vi "calc_phasemap_from_stored_images_ec.vi"() -> ()   [LabVIEW 2011]
uses:
  global_vars.vi
  <userlib>/_OpenG.lib/file/file.llb/Build Path - Traditional__ogtk.vi
panel:
  out "Intensity Graph":dbl[][](graph)
  out "u8_ar_phase map 2":u8[][](array[numeric])
  out "df_ar_unwrapped_px_ar 2":dbl[][](array[numeric])
  out "df_ar_unwrapped_px_ar":dbl[][](array[numeric])
  in  "current image 3":string="fringe2"
  out "difference":T1(plugin-control)
  out "Ndist_img":u8[][][](array[numeric])
  in  "read files no-dist":bool
  in  "normalize":bool
  out "Phase Line (unwrapped)":dbl[](graph)=[64.0, 65.0, 66.0, 68.0, 69.0, 70.0, 71.0, 73.0, 74.0, 75.0, 77.0, 78.0, 79.0, 80.0, 81.0, 83.0, 84.0, 85.0, 87.0, 88.0, 89.0, 90.0, 92.0, 93.0, 95.0, 96.0, 97.0, 98.0, 99.0, 101.0, 102.0, 103.0, 104.0, 106.0, 107.0, 108.0, 110.0, 111.0, 112.0, 114.0, 115.0, 116.0, 117.0, 119.0, 120.0, 121.0, 122.0, 124.0, 125.0, 126.0, 128.0, 129.0, 130.0, 131.0, 133.0, 134.0, 135.0, 136.0, 138.0, 139.0, 140.0, 141.0, 143.0, 144.0, 145.0, 147.0, 148.0, 149.0, 151.0, 152.0, 153.0, 154.0, 156.0, 157.0, 158.0, 159.0, 160.0, 162.0, 163.0, 165.0, 166.0, 167.0, 168.0, 170.0, 171.0, 172.0, 174.0, 175.0, 176.0, 177.0, 178.0, 180.0, 181.0, 182.0, 184.0, 185.0, 186.0, 187.0, 189.0, 190.0, 191.0, 193.0, 194.0, 195.0, 196.0, 198.0, 199.0, 200.0, 201.0, 203.0, 204.0, 205.0, 207.0, 208.0, 209.0, 210.0, 212.0, 213.0, 214.0, 215.0, 217.0, 218.0, 219.0, 221.0, 222.0, 223.0, 224.0, 226.0, 227.0, 228.0, 230.0, 231.0, 232.0, 233.0, 234.0, 236.0, 237.0, 238.0, 240.0, 241.0, 242.0, 243.0, 245.0, 246.0, 247.0, 249.0, 250.0, 251.0, 252.0, 254.0, 254.0, 255.0, 257.0, 258.0, 259.0, 260.0, 262.0, 263.0, 264.0, 266.0, 267.0, 268.0, 269.0, 271.0, 272.0, 273.0, 275.0, 276.0, 277.0, 278.0, 279.0, 281.0, 282.0, 283.0, 285.0, 286.0, 287.0, 288.0, 290.0, 291.0, 292.0, 294.0, 295.0, 296.0, 297.0, 299.0, 300.0, 301.0, 302.0, 304.0, 305.0, 306.0, 308.0, 309.0, 310.0, 311.0, 313.0, 314.0, 315.0, 316.0, 318.0, 319.0, 320.0, 322.0, 323.0, 324.0, 325.0, 327.0, 328.0, 329.0, 331.0, 332.0, 333.0, 334.0, 335.0, 337.0, 338.0, 339.0, 341.0, 342.0, 343.0, 344.0, 346.0, 347.0, 349.0, 350.0, 351.0, 352.0, 353.0, 355.0, 356.0, 357.0, 358.0, 360.0, 361.0, 362.0, 364.0, 365.0, 366.0, 368.0, 369.0, 370.0, 371.0, 373.0, 374.0, 375.0, 376.0, 378.0, 379.0, 380.0, 382.0, 383.0, 384.0, 385.0, 387.0, 388.0, 389.0, 390.0, 392.0, 393.0, 394.0, 395.0, 397.0, 398.0, 399.0, 401.0, 402.0, 403.0, 405.0, 406.0, 407.0, 408.0, 410.0, 411.0, 412.0, 413.0, 414.0, 416.0, 417.0, 419.0, 420.0, 421.0, 422.0, 424.0, 425.0, 426.0, 428.0, 429.0, 430.0, 431.0, 432.0, 434.0, 435.0, 436.0, 438.0, 439.0, 440.0, 441.0, 443.0, 444.0, 445.0, 447.0, 448.0, 449.0, 450.0, 452.0, 453.0, 454.0, 455.0, 457.0, 458.0, 459.0, 461.0, 462.0, 463.0, 464.0, 466.0, 467.0, 468.0, 469.0, 471.0, 472.0, 473.0, 475.0, 476.0, 477.0, 478.0, 480.0, 481.0, 482.0, 484.0, 485.0, 486.0, 487.0, 488.0, 490.0, 491.0, 492.0, 494.0, 495.0, 496.0, 497.0, 499.0, 500.0, 501.0, 503.0, 504.0, 505.0, 506.0, 508.0, 508.0, 509.0, 511.0, 512.0, 513.0, 514.0, 516.0, 517.0, 518.0, 520.0, 521.0, 522.0, 523.0, 525.0, 526.0, 527.0, 529.0, 530.0, 531.0, 532.0, 533.0, 535.0, 536.0, 537.0, 539.0, 540.0, 541.0, 542.0, 544.0, 545.0, 546.0, 548.0, 549.0, 550.0, 551.0, 553.0, 554.0, 555.0, 556.0, 558.0, 559.0, 560.0, 562.0, 563.0, 564.0, 565.0, 567.0, 568.0, 569.0, 570.0, 572.0, 573.0, 574.0, 576.0, 577.0, 578.0, 579.0, 581.0, 582.0, 583.0, 585.0, 586.0, 587.0, 588.0, 589.0, 591.0, 592.0, 593.0, 595.0, 596.0, 597.0, 598.0, 600.0, 601.0, 603.0, 604.0, 605.0, 606.0, 607.0, 609.0, 610.0, 611.0, 612.0, 614.0, 615.0, 616.0, 618.0, 619.0, 620.0, 622.0, 623.0, 624.0, 625.0, 627.0, 628.0, 629.0, 630.0, 632.0, 633.0, 634.0, 636.0, 637.0, 638.0, 639.0, 641.0, 642.0, 643.0, 644.0, 646.0, 647.0, 648.0, 649.0, 651.0, 652.0, 653.0, 655.0, 656.0, 657.0, 659.0, 660.0, 661.0, 662.0, 664.0, 665.0, 666.0, 667.0, 668.0, 670.0, 671.0, 673.0, 674.0, 675.0, 676.0, 678.0, 679.0, 680.0, 682.0, 683.0, 684.0, 685.0, 686.0, 688.0, 689.0, 690.0, 692.0, 693.0, 694.0, 695.0, 697.0, 698.0, 699.0, 701.0, 702.0, 703.0, 704.0, 706.0, 707.0, 708.0, 709.0, 711.0, 712.0, 713.0, 715.0, 716.0, 717.0, 718.0, 720.0, 721.0, 722.0, 723.0, 725.0, 726.0, 727.0, 729.0, 730.0, 731.0, 732.0, 734.0, 735.0, 736.0, 738.0, 739.0, 740.0, 741.0, 742.0, 744.0, 745.0, 746.0, 748.0, 749.0, 750.0, 751.0, 753.0, 754.0, 755.0, 757.0, 758.0, 759.0, 760.0, 762.0, 762.0, 763.0, 765.0, 766.0, 767.0, 768.0, 770.0, 771.0, 772.0, 774.0, 775.0, 776.0, 777.0, 779.0, 780.0, 781.0, 783.0, 784.0, 785.0, 786.0, 787.0, 789.0, 790.0, 791.0, 793.0, 794.0, 795.0, 796.0, 798.0, 799.0, 800.0, 802.0, 803.0, 804.0, 805.0, 807.0, 808.0, 809.0, 810.0, 812.0, 813.0, 814.0, 816.0, 817.0, 818.0, 819.0, 821.0, 822.0, 823.0, 824.0, 826.0, 827.0, 828.0, 830.0, 831.0, 832.0, 833.0, 835.0, 836.0, 837.0, 839.0, 840.0, 841.0, 842.0, 843.0, 845.0, 846.0, 847.0, 849.0, 850.0, 851.0, 852.0, 854.0, 855.0, 857.0, 858.0, 859.0, 860.0, 861.0, 863.0, 864.0, 865.0, 866.0, 868.0, 869.0, 870.0, 872.0, 873.0, 874.0, 876.0, 877.0, 878.0, 879.0, 881.0, 882.0, 883.0, 884.0, 886.0, 887.0, 888.0, 890.0, 891.0, 892.0, 893.0, 895.0, 896.0, 897.0, 898.0, 900.0, 901.0, 902.0, 903.0, 905.0, 906.0, 907.0, 909.0, 910.0, 911.0, 913.0, 914.0, 915.0, 916.0, 918.0, 919.0, 920.0, 921.0, 922.0, 924.0, 925.0, 927.0, 928.0, 929.0, 930.0, 932.0, 933.0, 934.0, 936.0, 937.0, 938.0, 939.0, 940.0, 942.0, 943.0, 944.0, 946.0, 947.0, 948.0, 949.0, 951.0, 952.0, 953.0, 955.0, 956.0, 957.0, 958.0, 960.0, 961.0, 962.0, 963.0, 965.0, 966.0, 967.0, 969.0, 970.0, 971.0, 972.0, 974.0, 975.0, 976.0, 977.0, 979.0, 980.0, 981.0, 983.0, 984.0, 985.0, 986.0, 988.0, 989.0, 990.0, 992.0, 993.0, 994.0, 995.0, 996.0, 998.0, 999.0, 1000.0, 1002.0, 1003.0, 1004.0, 1005.0, 1007.0, 1008.0, 1009.0, 1011.0, 1012.0, 1013.0, 1014.0, 1016.0, 1016.0, 1017.0, 1019.0, 1020.0, 1021.0, 1022.0, 1024.0, 1025.0, 1026.0, 1028.0, 1029.0, 1030.0, 1031.0, 1033.0, 1034.0, 1035.0, 1037.0, 1038.0, 1039.0, 1040.0, 1041.0, 1043.0, 1044.0, 1045.0, 1047.0, 1048.0, 1049.0, 1050.0, 1052.0, 1053.0, 1054.0, 1056.0, 1057.0, 1058.0, 1059.0, 1061.0, 1062.0, 1063.0, 1064.0, 1066.0, 1067.0, 1068.0, 1070.0, 1071.0, 1072.0, 1073.0, 1075.0, 1076.0, 1077.0, 1078.0, 1080.0, 1081.0, 1082.0, 1084.0, 1085.0, 1086.0, 1087.0, 1089.0, 1090.0, 1091.0, 1093.0, 1094.0, 1095.0, 1096.0, 1097.0, 1099.0, 1100.0, 1101.0, 1103.0, 1104.0, 1105.0, 1106.0, 1108.0, 1109.0, 1111.0, 1112.0, 1113.0, 1114.0, 1115.0, 1117.0, 1118.0, 1119.0, 1120.0, 1122.0, 1123.0, 1124.0, 1126.0, 1127.0, 1128.0, 1130.0, 1131.0, 1132.0, 1133.0, 1135.0, 1136.0, 1137.0, 1138.0, 1140.0, 1141.0, 1142.0, 1144.0, 1145.0, 1146.0, 1147.0, 1149.0, 1150.0, 1151.0, 1152.0, 1154.0, 1155.0, 1156.0, 1157.0, 1159.0, 1160.0, 1161.0, 1163.0, 1164.0, 1165.0, 1167.0, 1168.0, 1169.0, 1170.0, 1172.0, 1173.0, 1174.0, 1175.0, 1176.0, 1178.0, 1179.0, 1181.0, 1182.0, 1183.0, 1184.0, 1186.0, 1187.0, 1188.0, 1190.0, 1191.0, 1192.0, 1193.0, 1194.0, 1196.0, 1197.0, 1198.0, 1200.0, 1201.0, 1202.0, 1203.0, 1205.0, 1206.0, 1207.0, 1209.0, 1210.0, 1211.0, 1212.0, 1214.0, 1215.0, 1216.0, 1217.0, 1219.0, 1220.0, 1221.0, 1223.0, 1224.0, 1225.0, 1226.0, 1228.0, 1229.0, 1230.0, 1231.0, 1233.0, 1234.0, 1235.0, 1237.0, 1238.0, 1239.0, 1240.0, 1242.0, 1243.0, 1244.0, 1246.0, 1247.0, 1248.0, 1249.0, 1250.0, 1252.0, 1253.0, 1254.0, 1256.0, 1257.0, 1258.0, 1259.0, 1261.0, 1262.0, 1263.0, 1265.0, 1266.0, 1267.0, 1268.0, 1270.0, 1270.0, 1271.0, 1273.0, 1274.0, 1275.0, 1276.0, 1278.0, 1279.0, 1280.0, 1282.0, 1283.0, 1284.0, 1285.0, 1287.0, 1288.0, 1289.0, 1291.0, 1292.0, 1293.0, 1294.0, 1295.0, 1297.0, 1298.0, 1299.0, 1301.0, 1302.0, 1303.0, 1304.0, 1306.0, 1307.0, 1308.0, 1310.0, 1311.0, 1312.0, 1313.0, 1315.0, 1316.0, 1317.0, 1318.0, 1320.0, 1321.0, 1322.0, 1324.0, 1325.0, 1326.0, 1327.0, 1329.0, 1330.0, 1331.0, 1332.0]
  out "unwrapped phase map":T1(plugin-control)
  out "u8_ar_phase map":u8[][](array[numeric])
  out "Phase Line (wrapped)":u8[](graph)=[64, 65, 66, 68, 69, 70, 71, 73, 74, 75, 77, 78, 79, 80, 81, 83, 84, 85, 87, 88, 89, 90, 92, 93, 95, 96, 97, 98, 99, 101, 102, 103, 104, 106, 107, 108, 110, 111, 112, 114, 115, 116, 117, 119, 120, 121, 122, 124, 125, 126, 128, 129, 130, 131, 133, 134, 135, 136, 138, 139, 140, 141, 143, 144, 145, 147, 148, 149, 151, 152, 153, 154, 156, 157, 158, 159, 160, 162, 163, 165, 166, 167, 168, 170, 171, 172, 174, 175, 176, 177, 178, 180, 181, 182, 184, 185, 186, 187, 189, 190, 191, 193, 194, 195, 196, 198, 199, 200, 201, 203, 204, 205, 207, 208, 209, 210, 212, 213, 214, 215, 217, 218, 219, 221, 222, 223, 224, 226, 227, 228, 230, 231, 232, 233, 234, 236, 237, 238, 240, 241, 242, 243, 245, 246, 247, 249, 250, 251, 252, 254, 0, 1, 3, 4, 5, 6, 8, 9, 10, 12, 13, 14, 15, 17, 18, 19, 21, 22, 23, 24, 25, 27, 28, 29, 31, 32, 33, 34, 36, 37, 38, 40, 41, 42, 43, 45, 46, 47, 48, 50, 51, 52, 54, 55, 56, 57, 59, 60, 61, 62, 64, 65, 66, 68, 69, 70, 71, 73, 74, 75, 77, 78, 79, 80, 81, 83, 84, 85, 87, 88, 89, 90, 92, 93, 95, 96, 97, 98, 99, 101, 102, 103, 104, 106, 107, 108, 110, 111, 112, 114, 115, 116, 117, 119, 120, 121, 122, 124, 125, 126, 128, 129, 130, 131, 133, 134, 135, 136, 138, 139, 140, 141, 143, 144, 145, 147, 148, 149, 151, 152, 153, 154, 156, 157, 158, 159, 160, 162, 163, 165, 166, 167, 168, 170, 171, 172, 174, 175, 176, 177, 178, 180, 181, 182, 184, 185, 186, 187, 189, 190, 191, 193, 194, 195, 196, 198, 199, 200, 201, 203, 204, 205, 207, 208, 209, 210, 212, 213, 214, 215, 217, 218, 219, 221, 222, 223, 224, 226, 227, 228, 230, 231, 232, 233, 234, 236, 237, 238, 240, 241, 242, 243, 245, 246, 247, 249, 250, 251, 252, 254, 0, 1, 3, 4, 5, 6, 8, 9, 10, 12, 13, 14, 15, 17, 18, 19, 21, 22, 23, 24, 25, 27, 28, 29, 31, 32, 33, 34, 36, 37, 38, 40, 41, 42, 43, 45, 46, 47, 48, 50, 51, 52, 54, 55, 56, 57, 59, 60, 61, 62, 64, 65, 66, 68, 69, 70, 71, 73, 74, 75, 77, 78, 79, 80, 81, 83, 84, 85, 87, 88, 89, 90, 92, 93, 95, 96, 97, 98, 99, 101, 102, 103, 104, 106, 107, 108, 110, 111, 112, 114, 115, 116, 117, 119, 120, 121, 122, 124, 125, 126, 128, 129, 130, 131, 133, 134, 135, 136, 138, 139, 140, 141, 143, 144, 145, 147, 148, 149, 151, 152, 153, 154, 156, 157, 158, 159, 160, 162, 163, 165, 166, 167, 168, 170, 171, 172, 174, 175, 176, 177, 178, 180, 181, 182, 184, 185, 186, 187, 189, 190, 191, 193, 194, 195, 196, 198, 199, 200, 201, 203, 204, 205, 207, 208, 209, 210, 212, 213, 214, 215, 217, 218, 219, 221, 222, 223, 224, 226, 227, 228, 230, 231, 232, 233, 234, 236, 237, 238, 240, 241, 242, 243, 245, 246, 247, 249, 250, 251, 252, 254, 0, 1, 3, 4, 5, 6, 8, 9, 10, 12, 13, 14, 15, 17, 18, 19, 21, 22, 23, 24, 25, 27, 28, 29, 31, 32, 33, 34, 36, 37, 38, 40, 41, 42, 43, 45, 46, 47, 48, 50, 51, 52, 54, 55, 56, 57, 59, 60, 61, 62, 64, 65, 66, 68, 69, 70, 71, 73, 74, 75, 77, 78, 79, 80, 81, 83, 84, 85, 87, 88, 89, 90, 92, 93, 95, 96, 97, 98, 99, 101, 102, 103, 104, 106, 107, 108, 110, 111, 112, 114, 115, 116, 117, 119, 120, 121, 122, 124, 125, 126, 128, 129, 130, 131, 133, 134, 135, 136, 138, 139, 140, 141, 143, 144, 145, 147, 148, 149, 151, 152, 153, 154, 156, 157, 158, 159, 160, 162, 163, 165, 166, 167, 168, 170, 171, 172, 174, 175, 176, 177, 178, 180, 181, 182, 184, 185, 186, 187, 189, 190, 191, 193, 194, 195, 196, 198, 199, 200, 201, 203, 204, 205, 207, 208, 209, 210, 212, 213, 214, 215, 217, 218, 219, 221, 222, 223, 224, 226, 227, 228, 230, 231, 232, 233, 234, 236, 237, 238, 240, 241, 242, 243, 245, 246, 247, 249, 250, 251, 252, 254, 0, 1, 3, 4, 5, 6, 8, 9, 10, 12, 13, 14, 15, 17, 18, 19, 21, 22, 23, 24, 25, 27, 28, 29, 31, 32, 33, 34, 36, 37, 38, 40, 41, 42, 43, 45, 46, 47, 48, 50, 51, 52, 54, 55, 56, 57, 59, 60, 61, 62, 64, 65, 66, 68, 69, 70, 71, 73, 74, 75, 77, 78, 79, 80, 81, 83, 84, 85, 87, 88, 89, 90, 92, 93, 95, 96, 97, 98, 99, 101, 102, 103, 104, 106, 107, 108, 110, 111, 112, 114, 115, 116, 117, 119, 120, 121, 122, 124, 125, 126, 128, 129, 130, 131, 133, 134, 135, 136, 138, 139, 140, 141, 143, 144, 145, 147, 148, 149, 151, 152, 153, 154, 156, 157, 158, 159, 160, 162, 163, 165, 166, 167, 168, 170, 171, 172, 174, 175, 176, 177, 178, 180, 181, 182, 184, 185, 186, 187, 189, 190, 191, 193, 194, 195, 196, 198, 199, 200, 201, 203, 204, 205, 207, 208, 209, 210, 212, 213, 214, 215, 217, 218, 219, 221, 222, 223, 224, 226, 227, 228, 230, 231, 232, 233, 234, 236, 237, 238, 240, 241, 242, 243, 245, 246, 247, 249, 250, 251, 252, 254, 0, 1, 3, 4, 5, 6, 8, 9, 10, 12, 13, 14, 15, 17, 18, 19, 21, 22, 23, 24, 25, 27, 28, 29, 31, 32, 33, 34, 36, 37, 38, 40, 41, 42, 43, 45, 46, 47, 48, 50, 51, 52, 54, 55, 56, 57, 59, 60, 61, 62]
  in  "pick row for\nphase line plot":i32(slide) min=0 scale=0.0..499.0
  in  "calculate \nphase map":bool
  out "img_phase map":T1(plugin-control)
  out "current image":T1(plugin-control)
  out "Dist_img":u8[][][](array[numeric])
  in  "current image":string="fringe"
  in  "pick input image":i32
  in  "phase map file name":string="orig.png"
  in  "EXP Folder Path":path=path "X:/Cloud Drives/Dropbox/Europhotonics/FringeMan/Image Storage/01_09/playing around" caption="Enter or select file path"
  in  "save phasemap":bool
  in  "read files":bool
  in  "Stop Button":bool
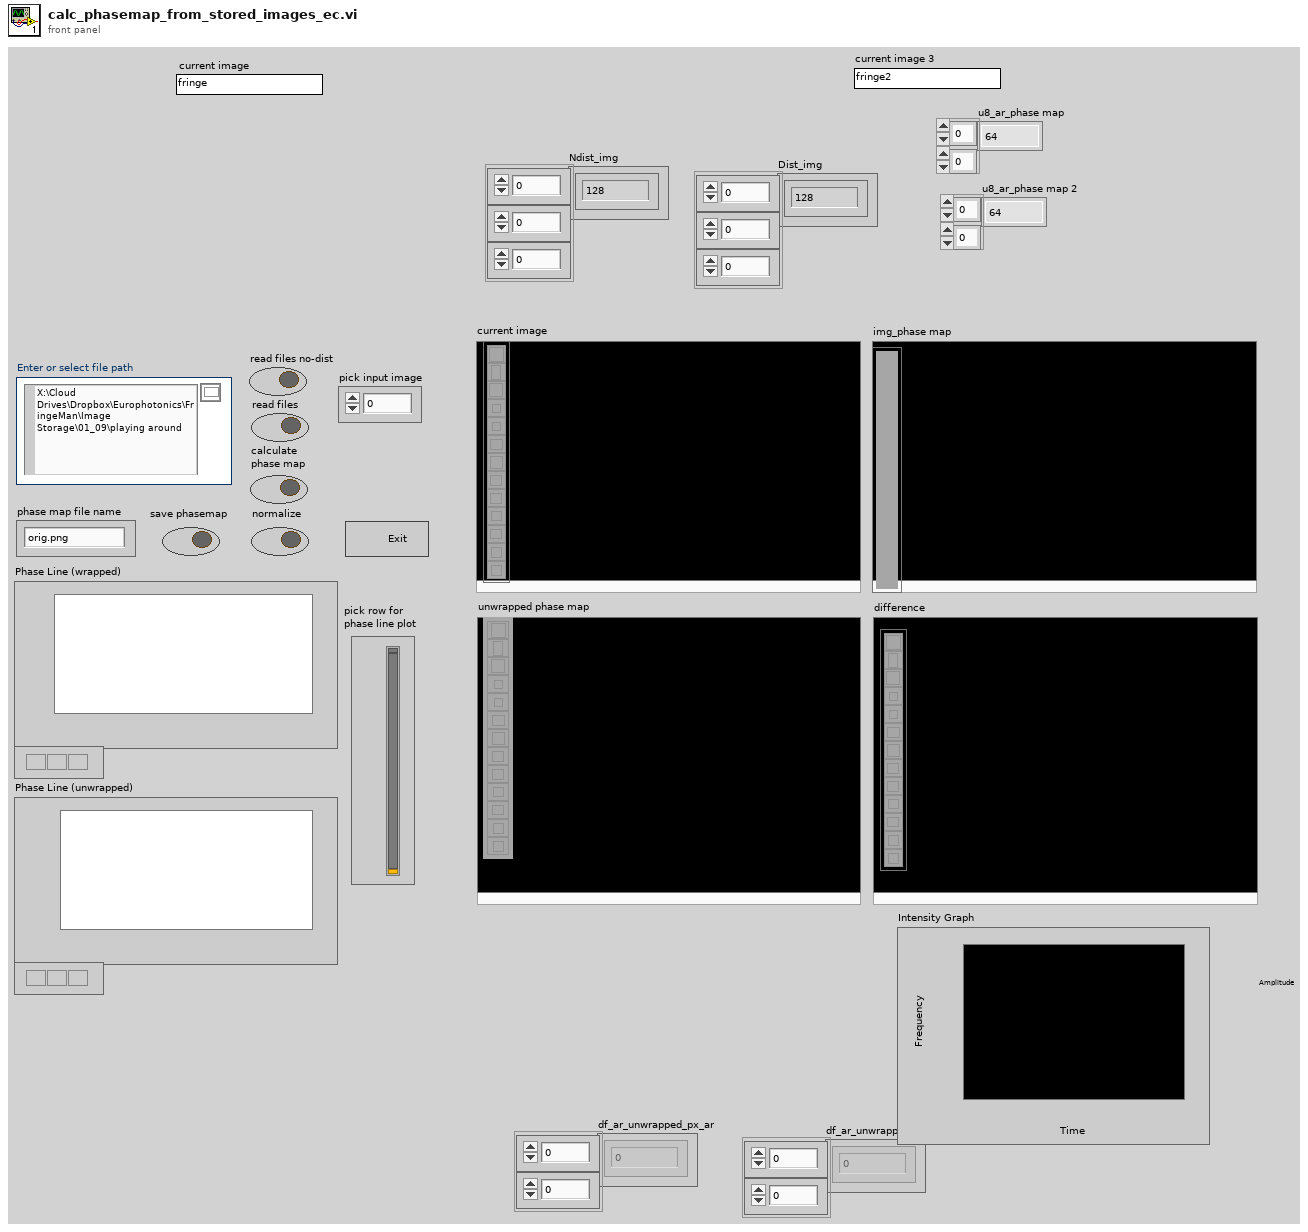
[diagram p1: front panel]
types:
  T1 = typedef "IMAQ Image.ctl" = refnum<image>
  T2 = typedef "Image Type" = u32
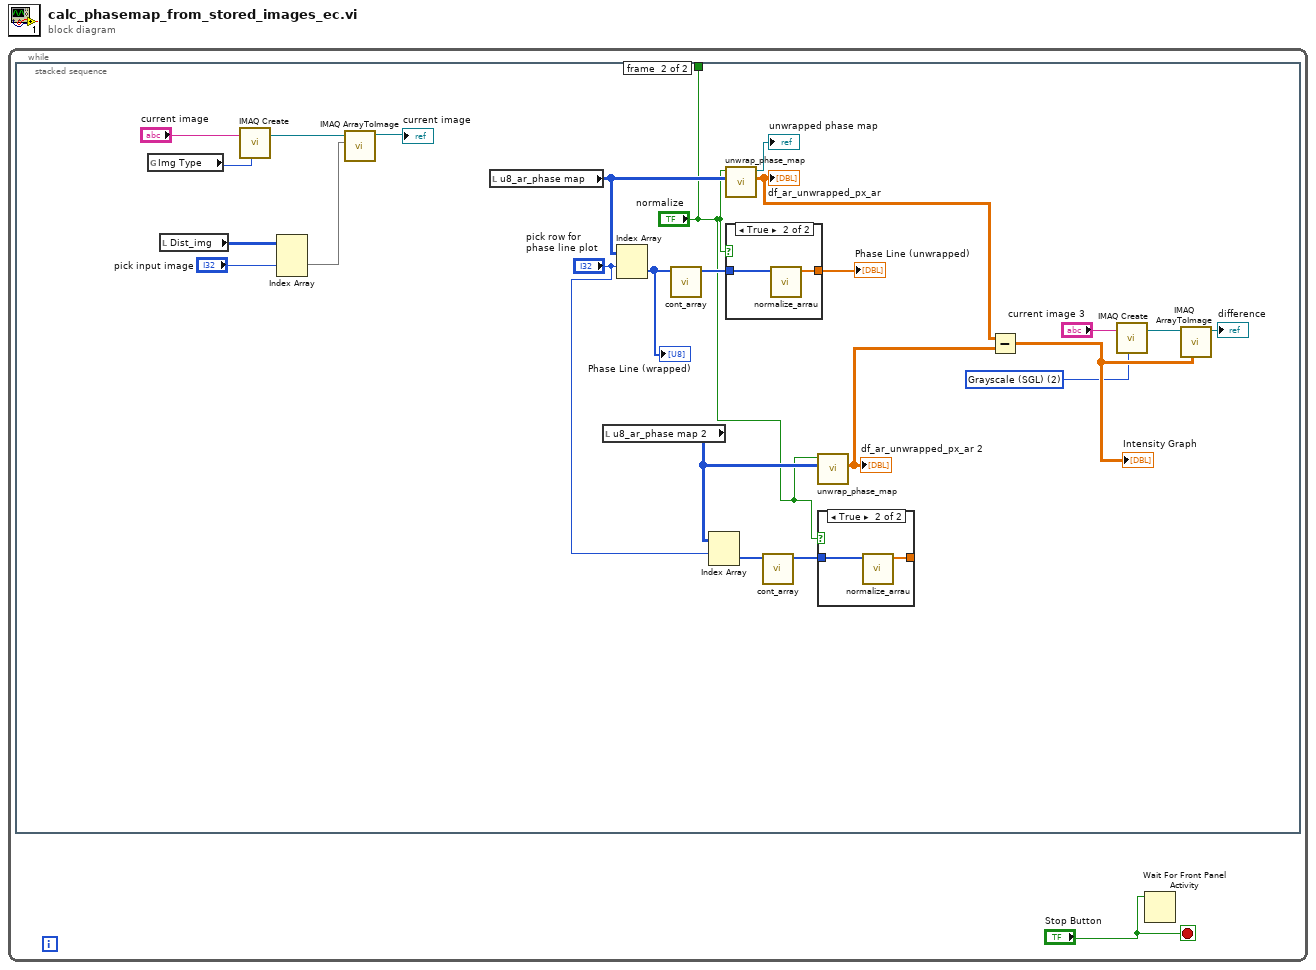
[diagram p0: block diagram]
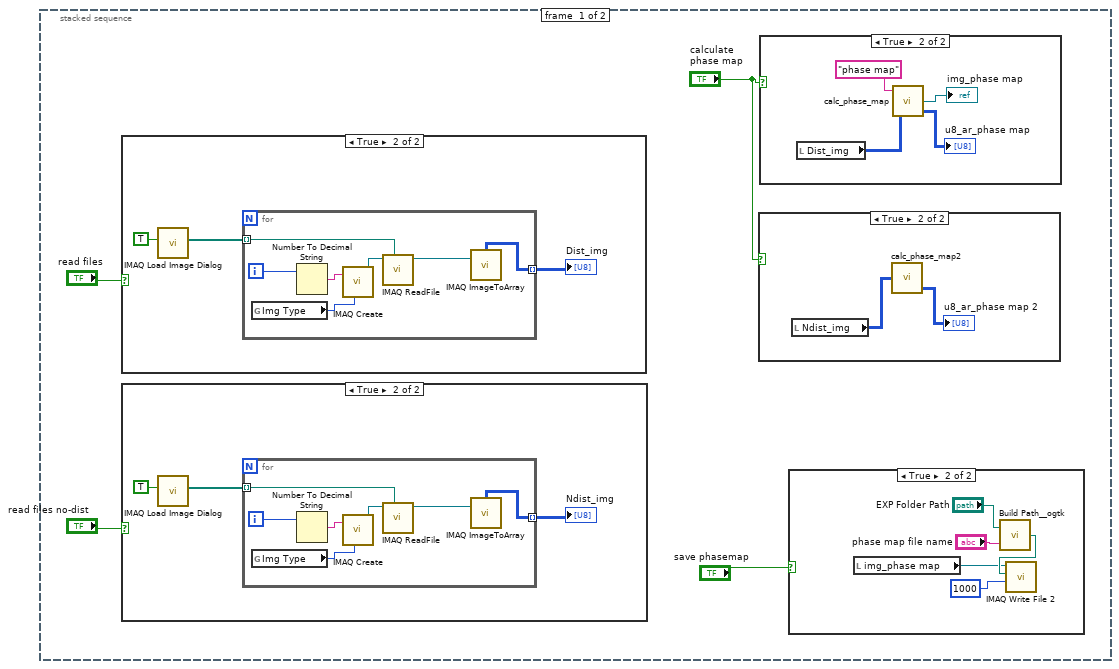
[diagram p2: hidden frame]
diagram:
  n1 = while {
    stop <- "Stop Button" stop-if-true
    n2 = stacked-sequence {
      tunnel: [_ "normalize"] -> _
      frame #0 {
        n3 = case shown="True" "read files" {
          frame False {
          }
          frame True {
            n4 = call "IMAQ Load Image Dialog"("Multiple Files? (No)"=TRUE) -> ("Paths"=w29:path[])  [unwired: 8 in, 2 out]
            n5 = for {
              tunnel: w29 -> [w36] mode=indexing
              tunnel: [w31] -> w27 mode=indexing
              i -> [w35]
              n6 = global read "global_vars.vi" "Img Type"() -> (w30:T2)
              n7 = Number To Decimal String(number=w35) -> (decimal integer string=w34:string)  [unwired: 1 in]
              n8 = call "IMAQ Create"("Image Name"=w34, "Image Type"=w30) -> ("New Image"=w33:T1)  [unwired: 2 in, 2 out]
              n9 = call "IMAQ ReadFile"("File Path"=w36, "Image"=w33) -> ("Image Out"=w32:T1)  [unwired: 5 in, 4 out]
              n10 = call "IMAQ ImageToArray"("Image"=w32) -> ("Image Pixels (U8)"=w31:u8[][])  [unwired: 3 in, 4 out]
            }
            "Dist_img" <- w27
          }
        }
        n11 = case shown="True" "read files no-dist" {
          frame False {
          }
          frame True {
            n12 = call "IMAQ Load Image Dialog"("Multiple Files? (No)"=TRUE) -> ("Paths"=w10:path[])  [unwired: 8 in, 2 out]
            n13 = for {
              tunnel: w10 -> [w17] mode=indexing
              tunnel: [w13] -> w8 mode=indexing
              i -> [w11]
              n14 = global read "global_vars.vi" "Img Type"() -> (w12:T2)
              n15 = Number To Decimal String(number=w11) -> (decimal integer string=w16:string)  [unwired: 1 in]
              n16 = call "IMAQ Create"("Image Name"=w16, "Image Type"=w12) -> ("New Image"=w15:T1)  [unwired: 2 in, 2 out]
              n17 = call "IMAQ ReadFile"("File Path"=w17, "Image"=w15) -> ("Image Out"=w14:T1)  [unwired: 5 in, 4 out]
              n18 = call "IMAQ ImageToArray"("Image"=w14) -> ("Image Pixels (U8)"=w13:u8[][])  [unwired: 3 in, 4 out]
            }
            "Ndist_img" <- w8
          }
        }
        n19 = case shown="True" "calculate \nphase map" {
          frame False {
          }
          frame True {
            n20 = local read "Ndist_img"() -> (w6:u8[][][])
            n21 = call "calc_phase_map2.vi"("u8_ar_image_pixel_array"=w6) -> ("raw phase map array"=→"u8_ar_phase map 2":u8[][])  [unwired: 4 in]
          }
        }
        n22 = case shown="True" "calculate \nphase map" {
          frame False {
          }
          frame True {
            n23 = local read "Dist_img"() -> (w20:u8[][][])
            n24 = call "calc_phase_map.vi"("u8_ar_image_pixel_array"=w20, "image name"="phase map" ("String")) -> ("raw phase map array"=→"u8_ar_phase map":u8[][], "phase map"=→"img_phase map":T1)  [unwired: 2 in]
          }
        }
        n25 = case shown="True" "save phasemap" {
          frame False {
          }
          frame True {
            n26 = local read "img_phase map"() -> (w22:T1)
            n27 = call-poly <userlib>:"Build Path__ogtk.vi"("name or relative path"="phase map file name", "base path"="EXP Folder Path") -> ("appended path"=w24:path)
            n28 = call-poly "IMAQ Write File 2"("Image Quality"=u32 1000, "File Path"=w24, "Image"=w22) -> ()  [unwired: 7 in, 2 out]
          }
        }
      }
      frame #1 {
        w37 = T2 2 items=["Grayscale (U8)", "Grayscale (I16)", "Grayscale (SGL)", "Complex (CSG)", "RGB (U32)", "HSL (U32)", "RGB (U64)", "Grayscale (U16)"] ("Image Type")
        n29 = global read "global_vars.vi" "Img Type"() -> (w57:T2)
        n30 = local read "Dist_img"() -> (w60:u8[][][])
        n31 = call "IMAQ Create"("Image Name"="current image", "Image Type"=w57) -> ("New Image"=w59:T1)  [unwired: 2 in, 2 out]
        n32 = Index Array(array=w60, index (dim 0)="pick input image") -> (element=w54:u8[][])  [unwired: 2 in]
        n33 = call "IMAQ ArrayToImage"("Image Pixels (U8)"=w54, "Image"=w59) -> ("Image Out"=→"current image":T1)  [unwired: 8 in, 1 out]
        n34 = local read "u8_ar_phase map"() -> (w52:u8[][])
        n35 = local read "u8_ar_phase map 2"() -> (w44:u8[][])
        n36 = Index Array(array=w52, index (row)="pick row for\nphase line plot") -> (element=w53:u8[])  [unwired: 1 in]
        "Phase Line (wrapped)" <- w53
        n37 = call "cont_array.vi"("u8_ar_phase map"=w53) -> ("Array"=w51:i16[])  [unwired: 10 in]
        n38 = Index Array(array=w44, index (row)="pick row for\nphase line plot") -> (element=w43:u8[])  [unwired: 1 in]
        n39 = call "unwrap_phase_map.vi"("u8_ar_phase map"=w52, "normalize (y)"="normalize") -> ("df_ar_unwrapped_px_ar"=w39:dbl[][], "Refnum out"=→"unwrapped phase map":T1)  [unwired: 8 in]
        "df_ar_unwrapped_px_ar" <- w39
        n40 = case shown="True" "normalize" {
          tunnel: w51 -> [w64 w66]
          tunnel: [w64 w65] -> w50
          frame False {
          }
          frame True {
            n41 = call "normalize_arrau.vi"("Array in"=w66) -> ("Array out"=w65:dbl[])  [unwired: 10 in]
          }
        }
        "Phase Line (unwrapped)" <- w50
        n42 = call "cont_array.vi"("u8_ar_phase map"=w43) -> ("Array"=w45:i16[])  [unwired: 10 in]
        n43 = call "unwrap_phase_map.vi"("u8_ar_phase map"=w44, "normalize (y)"="normalize") -> ("df_ar_unwrapped_px_ar"=w40:dbl[][])  [unwired: 8 in, 1 out]
        "df_ar_unwrapped_px_ar 2" <- w40
        n44 = case shown="True" "normalize" {
          tunnel: w45 -> [w61 w63]
          tunnel: [w61 w62] -> _
          frame False {
          }
          frame True {
            n45 = call "normalize_arrau.vi"("Array in"=w63) -> ("Array out"=w62:dbl[])  [unwired: 10 in]
          }
        }
        n46 = Subtract(x=w39, y=w40) -> (x-y=w38:dbl[][])
        "Intensity Graph" <- w38
        n47 = call "IMAQ Create"("Image Name"="current image 3", "Image Type"=w37) -> ("New Image"=w47:T1)  [unwired: 2 in, 2 out]
        n48 = call "IMAQ ArrayToImage"("Image Pixels (Float)"=w38, "Image"=w47) -> ("Image Out"=→"difference":T1)  [unwired: 8 in, 1 out]
      }
    }
    n49 = Wait For Front Panel Activity(3:"Stop Button") -> ()  [unwired: 2 in, 1 out]
  }
